vi "Execute Auto Charge Lo.vi"(0 "VISA resource name":refnum<visa-resource-name>, 11 "error in (no error)":errorcluster) -> (4 "VISA resource name out":refnum<visa-resource-name>, 15 "error out":errorcluster)   [LabVIEW 2016, in "eec EST 300.lvlib"]
doc: "SACG\nAutomatically Sets the Charge-LO parameter. This parameter is only available for the DCW or IR test types.\n\nThe cables and any test fixture should be connected before executing the command. The test parameters that are set for the step will be used when performing the auto setting. This command will perform an actual test and all safety precautions should be observed when using this command.\n\nThe Charge-LO function is used to check if the cables are connected properly at the beginning of a test."
uses:
  <instrlib>/eec EST 300/eec EST 300.lvlib
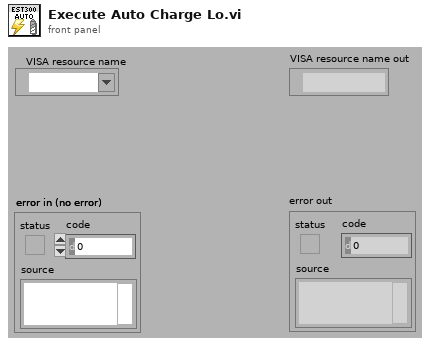
[diagram p1: front panel]
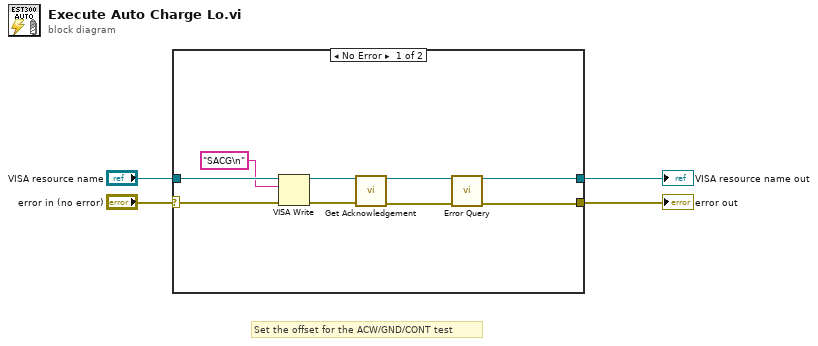
[diagram p0: block diagram]
diagram:
  # "Set the offset for the ACW/GND/CONT test"
  n1 = case shown="No Error" "error in (no error)" {
    selector: "error in (no error)" -> [w11 w15]
    tunnel: [w5 w15] -> w3
    tunnel: [w6 w14] -> w1
    tunnel: "VISA resource name" -> [w13 w14]
    frame No Error {
      n2 = VISA Write(VISA resource name=w13, write buffer="SACG\n" ("\"False\" Command"), error in (no error)=w11) -> (VISA resource name out=w10:refnum<visa-resource-name>, error out=w9:errorcluster)  [unwired: 1 out]
      n3 = call <instrlib>:"Get Acknowledgement.vi"("VISA resource name"=w10, "error in (no error)"=w9) -> ("VISA resource name out"=w8:refnum<visa-resource-name>, "error out"=w7:errorcluster)  [unwired: 12 in]
      n4 = call <instrlib>:"Error Query.vi"("VISA resource name"=w8, "error in (no error)"=w7) -> ("VISA resource name out"=w6:refnum<visa-resource-name>, "error out"=w5:errorcluster)  [unwired: 10 in, 2 out]
    }
    frame Error {
    }
  }
  "error out" <- w3
  "VISA resource name out" <- w1
